vi "Read File.vi"(8 "Error In":errorcluster, 10 "File":path=path "", 11 "KnownHosts In":refnum<class "Known Hosts.lvclass">) -> (0 "Error Out":errorcluster, 2 "Count":u64, 3 "KnownHosts Out":refnum<class "Known Hosts.lvclass">)   [LabVIEW 2018, in "Toolkit.lvlib" / "Known Hosts.lvclass"]
uses:
  Known Hosts.lvclass
  Known Hosts.lvclass/Known Hosts.ctl
  Session/Session.lvclass/Session.ctl
  SSH/SSH.lvclass/SSH.ctl
  Toolkit.lvlib
  Session/Session.lvclass
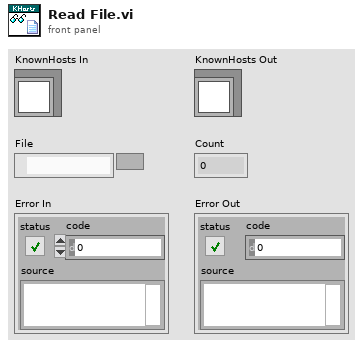
[diagram p1: front panel]
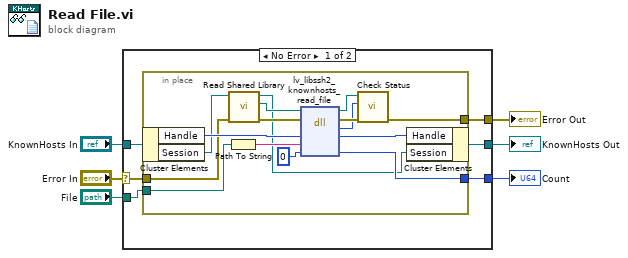
[diagram p0: block diagram]
diagram:
  n1 = case shown="No Error" "Error In" {
    selector: "Error In" -> [w10 w29]
    tunnel: "KnownHosts In" -> [w12 w28]
    tunnel: [w9 w29] -> w4
    tunnel: [w11 w28] -> w3
    tunnel: "File" -> [w8 _]
    tunnel: [w7 _] -> w1
    frame No Error {
      n2 = in-place {
        in-place-border: w10 -> [w18]
        in-place-border: [w23] -> w9
        in-place-border: w8 -> [w17]
        in-place-border: [w19] -> w7
        n3 = in-place-cluster #1(w12) -> ("Handle"=w27:u64, "Session"=w15:refnum<class "Session.lvclass">)
        n4 = Path To String(path=w17) -> (string=w21:string)
        n5 = call "Read Shared Library.vi"("Error In"=w18, "Session In"=w15) -> ("Erorr Out"=w16:errorcluster, "libssh2lv Shared Library"=w14:path, "Session Out"=w13:refnum<class "Session.lvclass">)  [unwired: 7 in]
        n6 = dll-call lib="D:/Users/cfield/Code/Field R&D Services/SSH/LV-LIBSSH2/LabVIEW/trunk/src/Toolkit/Support/lv-libssh2.*" fn="lv_libssh2_knownhosts_read_file"(path in=w14, error in=w16, "handle"=w27, "file"=w21, "count"=u64 0) -> (path out=w24:path, error out=w25:errorcluster, "status"=w22:i32, "handle"=w26:u64, "count"=w19:u64)  [unwired: 2 in]
        n7 = call "Check Status.vi"("Error In"=w25, "Status"=w22, "lv-libssh2 Shared Library In"=w24) -> ("Error Out"=w23:errorcluster)  [unwired: 7 in, 1 out]
        n8 = in-place-cluster #1("Handle"=w26, "Session"=w13) -> (w11:refnum<class "Known Hosts.lvclass">)
      }
    }
    frame Error {
    }
  }
  "Error Out" <- w4
  "KnownHosts Out" <- w3
  "Count" <- w1
